vi "Implement Authenticate.vi"(8 "error in (no error)":errorcluster, 10 "Challenge Dict":string, 11 "IAuthenticator in":refnum<class "IAuthenticator.lvclass">) -> (0 "error out":errorcluster, 1 "Authenticate Dict":string, 2 "Authenticate Signature":string, 3 "IAuthenticator out":refnum<class "IAuthenticator.lvclass">)   [LabVIEW 2020, in "wamplv.lvlib" / "IAuthenticator.lvclass"]
uses:
  IAuthenticator.lvclass
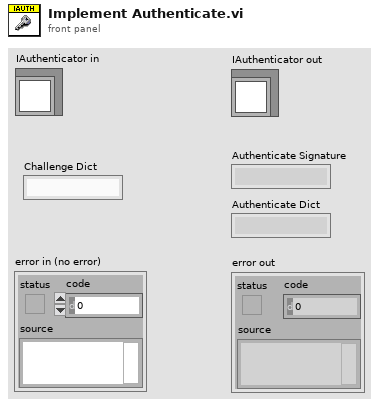
[diagram p1: front panel]
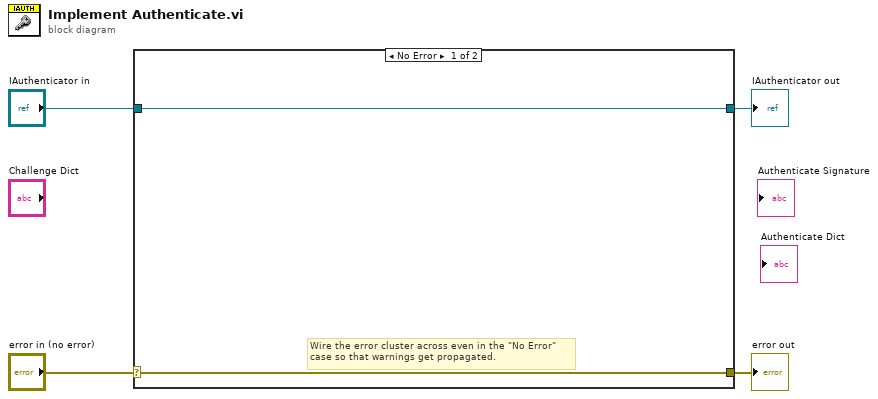
[diagram p0: block diagram]
diagram:
  n1 = case shown="No Error" "error in (no error)" {
    selector: "error in (no error)" -> [w5 w8]
    tunnel: [w5 w8] -> w3
    tunnel: [w6 w7] -> w1
    tunnel: "IAuthenticator in" -> [w6 w7]
    frame No Error {
      # "Wire the error cluster across even in the \"No Error\"\ncase so that warnings get propagated."
    }
    frame Error {
    }
  }
  "error out" <- w3
  "IAuthenticator out" <- w1
